vi "SwTmr Load Configuration Settings from XML.vi"(8 "error in (no error)":errorcluster, 11 "User Configuration in":T1={"Hardware Configuration"={"Physical Channel"="", "Maximum Input"=0.0, "Minimum Input"=0.0, "Sample Rate"=0.0, "Number of Samples"=0}, "Analysis Configuration"={"Statistics"=TRUE}, "New Data Behavior"=enum."Replace", "Time-Voltage transfer function file path (dialog if empty)"=path "", "Cell (V) Error Upper"=0.0, "Cell (V) Error Lower (type \"-\")"=0.0}) -> (0 "error out":errorcluster, 3 "User Configuration out":T1={"Hardware Configuration"={"Physical Channel"="", "Maximum Input"=0.0, "Minimum Input"=0.0, "Sample Rate"=0.0, "Number of Samples"=0}, "Analysis Configuration"={"Statistics"=TRUE}, "New Data Behavior"=enum."Replace", "Time-Voltage transfer function file path (dialog if empty)"=path "", "Cell (V) Error Upper"=0.0, "Cell (V) Error Lower (type \"-\")"=0.0})   [LabVIEW 2017]
doc: "Attempts to load previous user specified settings from an XML file.\n\nThis VI will not generate an error. If a suitable XML file can't be loaded and parsed then it will simply return the default settings."
uses:
  controls/SwTmr User Specified Data.ctl
  controls/SwTmr HW Configuration.ctl
  controls/SwTmr Analysis Configuration.ctl
  controls/SwTmr New Data Behavior.ctl
  controls/SwTmr Transfer Func File Path.ctl
  <vilib>/Utility/xml.llb/Read From XML File(string).vi
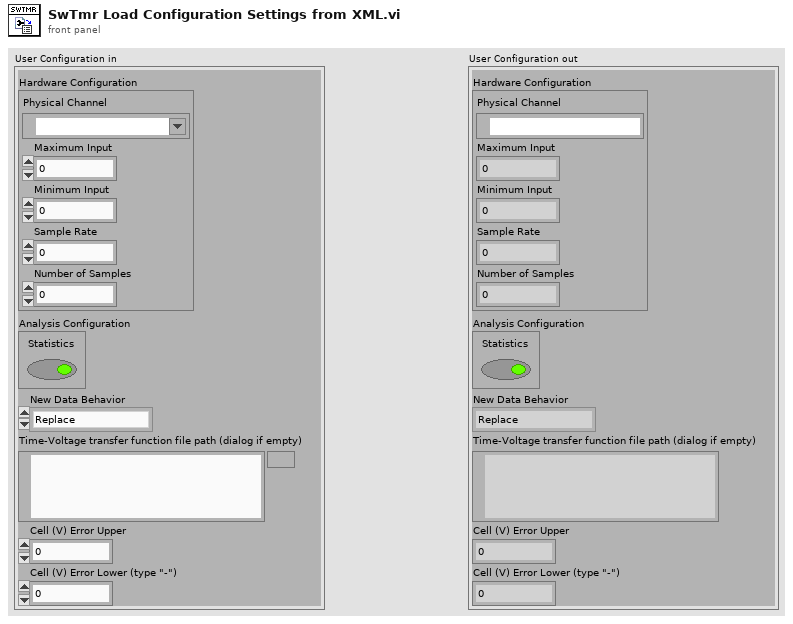
[diagram p1: front panel]
types:
  T1 = typedef "SwTmr User Specified Data.ctl" = cluster{"Hardware Configuration":T2, "Analysis Configuration":T3, "New Data Behavior":T4, "Time-Voltage transfer function file path (dialog if empty)":T5, "Cell (V) Error Upper":dbl, "Cell (V) Error Lower (type \"-\")":dbl}
  T2 = typedef "SwTmr HW Configuration.ctl" = cluster{"Physical Channel":tag, "Maximum Input":dbl, "Minimum Input":dbl, "Sample Rate":dbl, "Number of Samples":i32}
  T3 = typedef "SwTmr Analysis Configuration.ctl" = cluster{"Statistics":bool}
  T4 = typedef "SwTmr New Data Behavior.ctl" = enum16{"Replace", "Overlay", "Append"}
  T5 = typedef "SwTmr Transfer Func File Path.ctl" = path
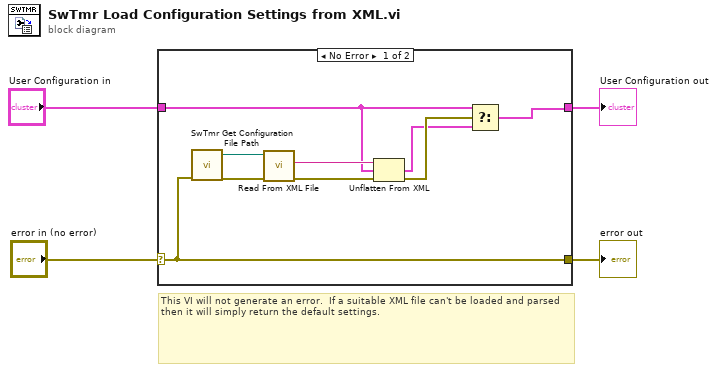
[diagram p0: block diagram]
diagram:
  # "This VI will not generate an error.  If a suitable XML file can't be loaded and parsed then it will simply return the default settings."
  n1 = case shown="No Error" "error in (no error)" {
    selector: "error in (no error)" -> [w10 w15]
    tunnel: [w10 w15] -> w3
    tunnel: "User Configuration in" -> [w7 w14]
    tunnel: [w5 w14] -> w1
    frame No Error {
      n2 = call "SwTmr Get Configuration File Path.vi"("error in (no error)"=w10) -> ("error out"=w12:errorcluster, "XML File Path"=w13:path)  [unwired: 9 in]
      n3 = call-poly <vilib>:"Read From XML File.vi"("error in (no error)"=w12, "XML File Path"=w13) -> ("error out"=w9:errorcluster, "XML Elements"=w11:string)  [unwired: 7 in, 1 out]
      n4 = Unflatten From XML(xml string=w11, type=w7, error in (no error)=w9) -> (value=w6:T1, error out=w8:errorcluster)
      n5 = Select(t=w7, s=w8, f=w6) -> (s? t:f=w5:T1)
    }
    frame Error {
    }
  }
  "error out" <- w3
  "User Configuration out" <- w1
